vi "Create DMA Buffers.vi"(8 "error in (no error)":errorcluster, 9 "Config":T2, 10 "TDMS DAQ in":refnum<class "TDMS DAQ.lvclass">, 11 "State In":T1) -> (0 "error out":errorcluster, 3 "State Out":T1)   [LabVIEW 2020, in "TDMS DAQ.lvlib" / "TDMS DAQ.lvclass"]
uses:
  TDMS DAQ.lvclass
  Configure TDMS DAQ.ctl
  Helper Loop State.ctl
  <vilib>/Natan Biesmans/G2CPU GPU and CPU HPC Toolkit/G2CPU Libraries/Async IO/DMA Manager/DMA Manager.lvclass
  TDMS DAQ.lvclass/TDMS DAQ.ctl
  fad5fc6d-ad9e-4e31-9e33-efe3a6be4393.vi
  fad5fc6d-ad9e-4e31-9e33-efe3a6be4393.vi/c1c6ba82-99b7-4273-a704-85eea64f3b4b.vi
  fad5fc6d-ad9e-4e31-9e33-efe3a6be4393.vi/fcfd33d5-6ac1-42cc-9267-61f2760a5aae.vi
  fad5fc6d-ad9e-4e31-9e33-efe3a6be4393.vi/8aa0c4af-4daa-4014-9a01-595272b02124.vi
  fad5fc6d-ad9e-4e31-9e33-efe3a6be4393.vi/6d883df8-3b64-4008-8da1-8b1f8b11b48b.vi
  fad5fc6d-ad9e-4e31-9e33-efe3a6be4393.vi/8aa0c4af-4daa-4014-9a01-595272b02124.vi/c174a7f7-781d-4fed-8bab-bf30bc03dac0.vi
  fad5fc6d-ad9e-4e31-9e33-efe3a6be4393.vi/6d883df8-3b64-4008-8da1-8b1f8b11b48b.vi/313ec8c5-c203-475c-9de0-0583f6fb8b4d.vi
  <vilib>/Natan Biesmans/G2CPU GPU and CPU HPC Toolkit/G2CPU Libraries/Arrays/1DArray/s16/1D Array s16.lvclass
  C:/Program Files/National Instruments/LabVIEW 2025/vi.lib/Natan Biesmans/G2CPU GPU and CPU HPC Toolkit/G2CPU Libraries/Arrays/Array/Array Prototype.lvclass
  <vilib>/Natan Biesmans/G2CPU GPU and CPU HPC Toolkit/G2CPU Libraries/Manage Environment/G2CPU Get Backend.vi
  <vilib>/Utility/error.llb/Error Cluster From Error Code.vi
  <vilib>/Natan Biesmans/G2CPU GPU and CPU HPC Toolkit/ArrayFire Driver/VIs/Run as Multi Device.vi
  <vilib>/Natan Biesmans/G2CPU GPU and CPU HPC Toolkit/G2CPU Libraries/Runtime Licensing/G2CPU License Check.vi
  <vilib>/Natan Biesmans/G2CPU GPU and CPU HPC Toolkit/G2CPU Libraries/Manage Environment/Find AF DLL.vi
  <vilib>/Natan Biesmans/G2CPU GPU and CPU HPC Toolkit/G2CPU Libraries/Arrays/Array/G2CPU Set Array Pointer.vi
  <resource>/Natan Biesmans/G2CPU GPU and CPU HPC Toolkit/Garbage Collector/G2CPU DMAGarbageCollectorFGV.vi
  <vilib>/Natan Biesmans/G2CPU GPU and CPU HPC Toolkit/G2CPU Libraries/Arrays/Array/Array Prototype.lvclass
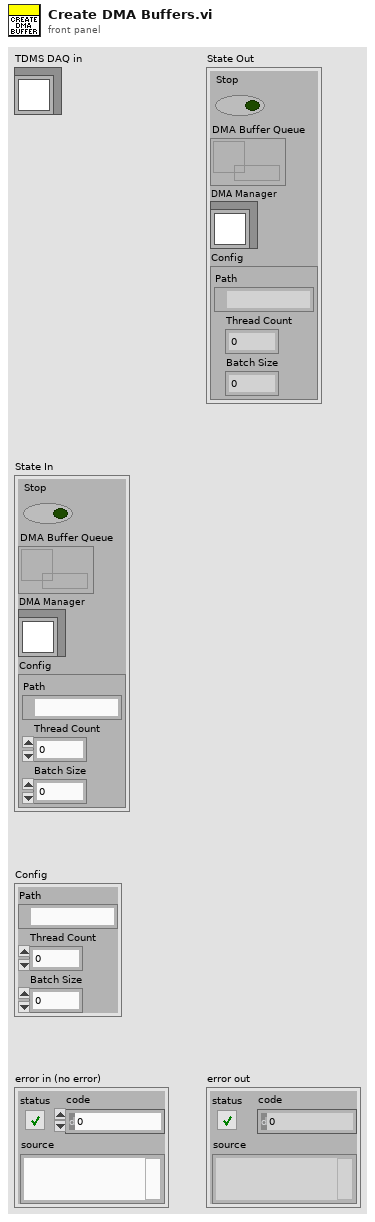
[diagram p1: front panel]
types:
  T1 = typedef "TDMS DAQ.lvlib/TDMS DAQ.lvclass/Helper Loop State.ctl" = cluster{"Stop":bool, "DMA Buffer Queue":refnum<queue>, "DMA Manager":refnum<class "DMA Manager.lvclass">, "Config":T2}
  T2 = typedef "TDMS DAQ.lvlib/TDMS DAQ.lvclass/Configure TDMS DAQ.ctl" = cluster{"Path":path, "Thread Count":i32, "Batch Size":i32}
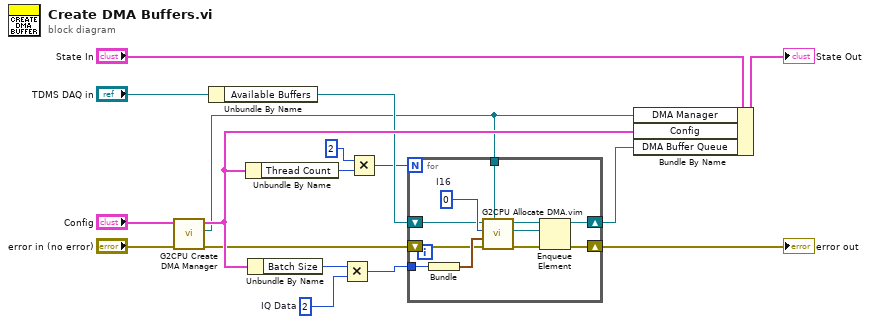
[diagram p0: block diagram]
diagram:
  w16 = 2  # IQ Data
  n1 = call <vilib>:"G2CPU Create DMA Manager.vi"("error in (no error)"="error in (no error)") -> ("error out"=w13:errorcluster, "DMA Manager"=w10:refnum<class "DMA Manager.lvclass">)  [unwired: 9 in]
  n2 = Unbundle By Name("TDMS DAQ in") -> ("Available Buffers"=w12:refnum<queue>)
  n3 = Unbundle By Name("Config") -> ("Thread Count"=w3:i32)
  n4 = Unbundle By Name("Config") -> ("Batch Size"=w1:i32)
  n5 = Multiply(x=w1, y=w16) -> (x*y=w15:i32)
  n6 = Multiply(x=2, y=w3) -> (x*y=w4:i32)
  n7 = for {
    N: w4 -> [_]
    tunnel: w10 -> [w26]
    tunnel: w15 -> [w23]
    shift-right: [w20] -> w2
    shift-left: w13 -> [w22]
    shift-right: [w19] -> w8
    shift-left: w12 -> [w18]
    w25 = i16 0  # I16
    n8 = Bundle(w23) -> (w24:cluster{i32})  [unwired: 1 in]
    n9 = call "G2CPU Allocate DMA.vim"("DMA Manager"=w26, "error in (no error)"=w22, "Size"=w24, "Datatype"=w25) -> ("error out"=w21:errorcluster, "DMA Memory"=w17:refnum<data-value>)  [unwired: 6 in]
    n10 = Enqueue Element(queue=w18, element=w17, error in (no error)=w21) -> (queue out=w19:refnum<queue>, error out=w20:errorcluster)  [unwired: 1 in, 1 out]
  }
  "error out" <- w2
  n11 = Bundle By Name(cluster="State In", "DMA Manager"=w10, "Config"="Config", "DMA Buffer Queue"=w8) -> (→"State Out":T1)
